vi "GetInputLabel.vi"(10 "Input Index":i32, 11 "Inputs":T1[](array[typedef])) -> (3 "Input Label":string)   [LabVIEW 2012, in "Virtual-PGA.lvlib"]
uses:
  Virtual-PGA.lvlib
  Public/Controls/Input.ctl
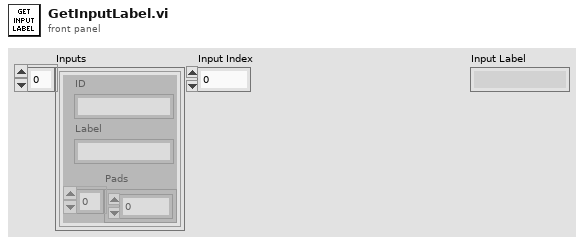
[diagram p1: front panel]
types:
  T1 = typedef "Virtual-PGA.lvlib/Input.ctl" = cluster{"ID":string, "Label":string, "Pads":u32[]}
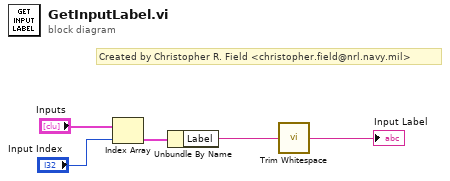
[diagram p0: block diagram]
diagram:
  # "Created by Christopher R. Field <christopher.field@nrl.navy.mil>"
  n1 = Index Array(array="Inputs", index="Input Index") -> (element=w3:T1)
  n2 = Unbundle By Name(w3) -> ("Label"=w2:string)
  n3 = call <vilib>:"Trim Whitespace.vi"("string"=w2) -> ("trimmed string"=→"Input Label":string)  [unwired: 1 in]
